vi "Configure CRDS.vi"(11 "Controller In":refnum<class "gController.lvclass">) -> ()   [LabVIEW 2016, in "Controller.lvlib" / "gController.lvclass"]
uses:
  gController.lvclass
  C:/Program Files (x86)/National Instruments/LabVIEW 2016/vi.lib/MSR Consulting, LLC/General Reuse/SuperActor/SuperActor.lvclass
  C:/Program Files (x86)/National Instruments/LabVIEW 2016/vi.lib/ActorFramework/Actor/Actor.lvclass
  Messages/Update CRD Laser Enable State MSG/Update CRD Laser Enable State MSG.lvclass
  G:/sw_repo/For Builds/Nicholas/Controller/Messages/Generic Boolean MSG/Generic Boolean Message.lvclass
  C:/Program Files (x86)/National Instruments/LabVIEW 2016/vi.lib/ActorFramework/Message/Message.lvclass
  Messages/Change Heater SP MSG/Change Heater SP MSG.lvclass
  Messages/Change Heater Ctl Params MSG/Change Heater Ctl Params.lvclass
  <vilib>/MSR Consulting, LLC/General Reuse/Session APIs/File Access/Config Data/Config Data.lvclass
  <vilib>/MSR Consulting, LLC/General Reuse/SuperActor/SuperActor.lvclass/SuperActor.ctl
  <vilib>/ActorFramework/Actor/Actor.lvclass/Actor.ctl
  <vilib>/ActorFramework/Message Enqueuer/Message Enqueuer.lvclass/Message Enqueuer.ctl
  <vilib>/MSR Consulting, LLC/General Reuse/Session APIs/File Access/Config Data/Config Data.lvclass/Config Data.ctl
  Messages/Change Heater Ctl Params MSG/Change Heater Ctl Params.lvclass/Change Heater Ctl Params.ctl
  Messages/Change Heater SP MSG/Change Heater SP MSG.lvclass/Change Heater SP MSG.ctl
  Messages/Generic Boolean MSG/Generic Boolean Message.lvclass/Generic Boolean Message.ctl
  <vilib>/MSR Consulting, LLC/General Reuse/SuperActor/Read Config Session.vi
  <vilib>/MSR Consulting, LLC/General Reuse/Session APIs/File Access/Config Data/Accessors/Read Ref.vi
  Messages/Change Heater Ctl Params MSG/Write id.vi
  Messages/Change Heater Ctl Params MSG/Write ctl.vi
  Messages/Generic Boolean MSG/Write Bool.vi
  Messages/Change Heater SP MSG/Write id.vi
  Messages/Change Heater SP MSG/Write sp.vi
  <vilib>/ActorFramework/Message Enqueuer/Init from Existing Queue.vi
  <vilib>/MSR Consulting, LLC/General Reuse/Session APIs/File Access/Config Data/Read Array/Read DBL Array.vi
  <vilib>/Utility/config.llb/Read Key (Double).vi
  <vilib>/Utility/config.llb/Read Key (Boolean).vi
  <vilib>/ActorFramework/Message Priority Queue/Priority Enqueue.vi
  <vilib>/MSR Consulting, LLC/General Reuse/Session APIs/_Session Fwk/Session - Root.lvclass
  <vilib>/ActorFramework/Message Enqueuer/Message Enqueuer.lvclass
  <vilib>/Utility/config.llb/NI_LVConfig.lvlib
  <vilib>/ActorFramework/Actor/Actor.lvclass
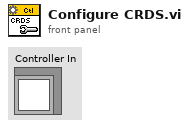
[diagram p1: front panel]
types:
  T1 = typedef "Session - Root.lvclass/Session Handle.ctl" = refnum<data-value>
  T2 = typedef "NI_LVConfig.lvlib/Config Data RefNum.ctl" = refnum<k1>
  T3 = cluster{"Read Array Data:DBL Data[0]":dbl, "Read Array Data:DBL Data[1]":dbl, "Read Array Data:DBL Data[2]":dbl}
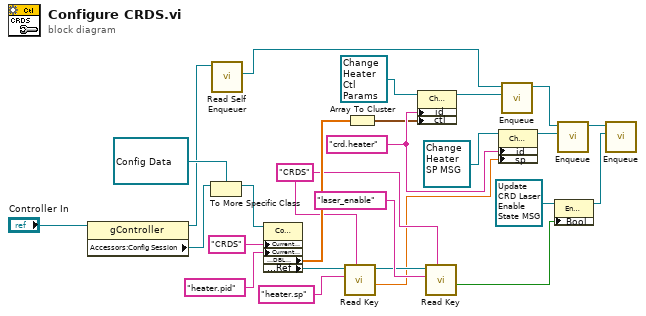
[diagram p0: block diagram]
diagram:
  w10 = "crd.heater" ("id")
  w14 = "CRDS" ("section")
  n1 = property class="gController"(reference="Controller In") -> (reference out=w3:refnum<class "gController.lvclass">, "Accessors:Config Session"=w5:T1)  [unwired: 1 in, 1 out]
  n2 = To More Specific Class(target class=refnum<data-value> refnum, reference=w5) -> (specific class reference=w1:refnum<data-value>)  [unwired: 1 in, 1 out]
  n3 = call <vilib>:"Read Self Enqueuer.vi"("Actor"=w3) -> ("Self Enqueuer"=w2:refnum<class "Message Enqueuer.lvclass">)  [unwired: 10 in]
  n4 = property class="Config Data"(reference=w1, "Current Section"="CRDS", "Current Key"="heater.pid") -> ("Read Array Data:DBL Data"=w21:dbl[], "Accessors:Ref"=w25:T2)  [unwired: 1 in, 2 out]
  n5 = call-poly <vilib>:"Read Key.vi"("section"=w14, "key"="heater.sp", "refnum"=w25) -> ("value"=w11:dbl, "refnum out"=w13:T2)  [unwired: 5 in, 2 out]
  n6 = Array To Cluster(array=w21) -> (cluster=w8:T3)
  n7 = property class="Change Heater Ctl Params"(reference=refnum<class "Change Heater Ctl Params.lvclass"> refnum ("Controller.lvlib:Change Heater Ctl Params"), "id"=w10, "ctl"=w8) -> (reference out=w9:refnum<class "Change Heater Ctl Params.lvclass">)  [unwired: 1 in, 1 out]
  n8 = call-poly <vilib>:"Read Key.vi"("section"=w14, "key"="laser_enable", "refnum"=w13) -> ("value"=w17:bool)  [unwired: 5 in, 3 out]
  n9 = property class="Change Heater SP MSG"(reference=refnum<class "Change Heater SP MSG.lvclass"> refnum ("Controller.lvlib:Change Heater SP MSG"), "id"=w10, "sp"=w11) -> (reference out=w12:refnum<class "Change Heater SP MSG.lvclass">)  [unwired: 1 in, 1 out]
  n10 = call <vilib>:"Enqueue.vi"("Message"=w9, "Message Enqueuer in"=w2) -> ("Message Enqueuer out"=w23:refnum<class "Message Enqueuer.lvclass">)  [unwired: 8 in, 1 out]
  n11 = property class="Enable CRD Laser MSG"(reference=refnum<class "Update CRD Laser Enable State MSG.lvclass"> refnum ("Controller.lvlib:Enable CRD Laser MSG"), "Bool"=w17) -> (reference out=w18:refnum<class "Update CRD Laser Enable State MSG.lvclass">)  [unwired: 1 in, 1 out]
  n12 = call <vilib>:"Enqueue.vi"("Message"=w12, "Message Enqueuer in"=w23) -> ("Message Enqueuer out"=w24:refnum<class "Message Enqueuer.lvclass">)  [unwired: 8 in, 1 out]
  n13 = call <vilib>:"Enqueue.vi"("Message"=w18, "Message Enqueuer in"=w24) -> ()  [unwired: 8 in, 2 out]
